vi "2_12.vi"() -> ()   [LabVIEW 2017]
panel:
  out "XY Graph":cluster{"Y":dbl[], "Y":dbl[]}[](graph)
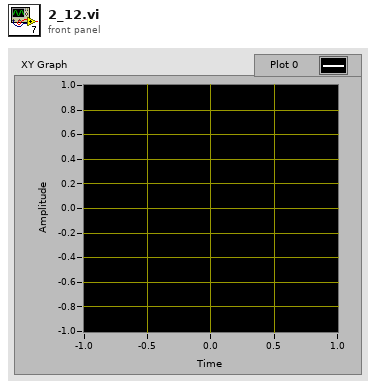
[diagram p1: front panel]
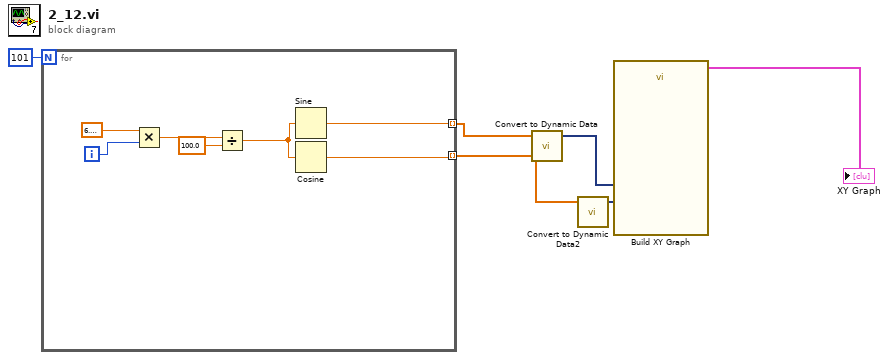
[diagram p0: block diagram]
diagram:
  n1 = for {
    N: 101 -> [_]
    tunnel: [w9] -> w4 mode=indexing
    tunnel: [w8] -> w2 mode=indexing
    i -> [w12]
    n2 = Multiply(x=6.283185307179586, y=w12) -> (x*y=w11:dbl)
    n3 = Divide(x=w11, y=100.0) -> (x/y=w7:dbl)
    n4 = Sine(x=w7) -> (sin(x)=w9:dbl)
    n5 = Cosine(x=w7) -> (cos(x)=w8:dbl)
  }
  n6 = call "Convert to Dynamic Data"("Array"=w4) -> ("Dynamic Data Type"=w3:dynamicdata)  [unwired: 3 in]
  n7 = call "Convert to Dynamic Data2"("Array"=w2) -> ("Dynamic Data Type"=w1:dynamicdata)  [unwired: 3 in]
  n8 = call "Build XY Graph"("Y Input"=w1, "X Input"=w3) -> ("XY Graph"=→"XY Graph":cluster{"X":dbl[], "Y":dbl[]}[])  [unwired: 8 in, 1 out]
